vi "Plot Euler Spiral.vi"() -> ()   [LabVIEW 2018]
panel:
  out "L2":dbl
  out "Normalized":cluster{"Time":dbl, "Length":dbl, "Radius":dbl}
  out "Scaled":cluster{"Time":dbl, "Length":dbl, "Radius":dbl}
  in  "Y Positive":bool=TRUE
  in  "X Positive":bool=TRUE
  out "Length to Vertex":dbl
  in  "Scale Mag":dbl(slide)=1.096774193548387 scale=0.0..10.0
  out "Tangent angle (deg)":dbl
  in  "Additional circle arc (rad)":dbl(slide) scale=0.0..3.0
  out "Tangent angle (rad)":dbl
  out "Tangent Point":cluster{dbl, dbl}
  in  "Steps":dbl=1000.0
  in  "T":dbl(slide)=0.6451612903225806 scale=0.0..2.0
  out "XY Graph":cluster{cluster{dbl, dbl}[]}[](graph)
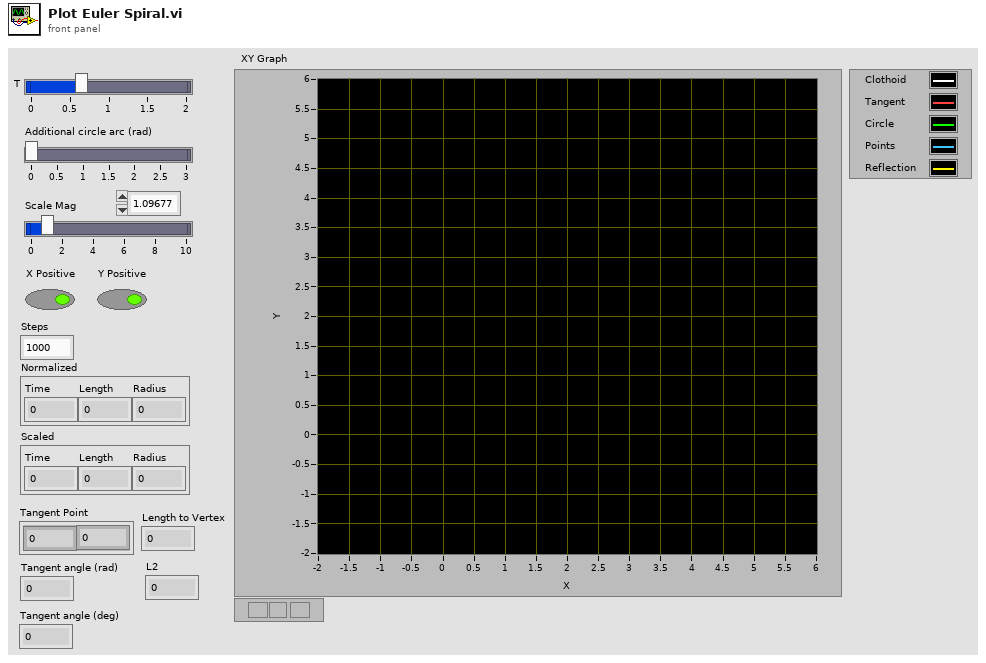
[diagram p1: front panel]
types:
  T1 = cluster{cluster{dbl, dbl}[], cluster{dbl, dbl}[], cluster{dbl, dbl}}
  T2 = cluster{"Negated Y":i32, "Scaled Sign Vector":cluster{"X":dbl, "Y":dbl}, "Combined":i32, "Additional circle arc (rad)":dbl}
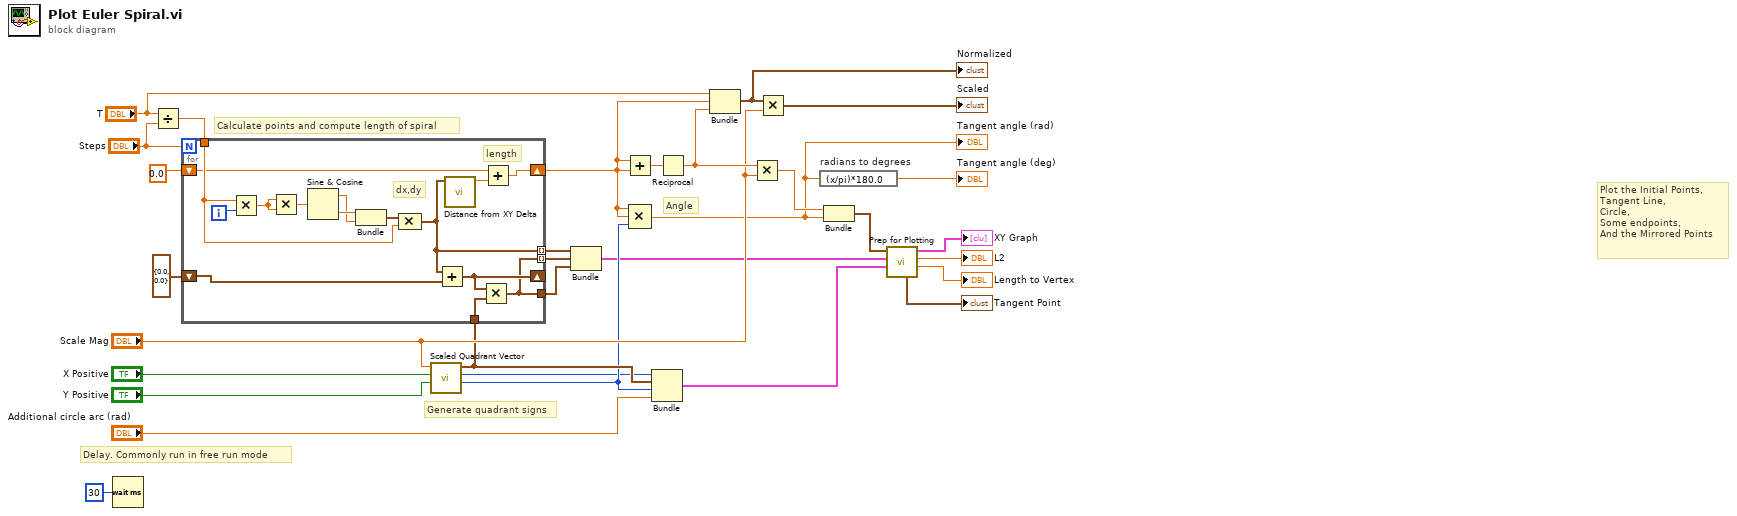
[diagram p0: block diagram]
diagram:
  # "Generate quadrant signs"
  # "Delay. Commonly run in free run mode"
  # "Plot the Initial Points,\nTangent Line,\nCircle,\nSome endpoints,\nAnd the Mirrored Points"
  # "Angle"
  # "Calculate points and compute length of spiral"
  n1 = Wait (ms)(milliseconds to wait=u32 30) -> ()  [unwired: 1 out]
  n2 = Divide(x="T", y="Steps") -> (x/y=w29:dbl)
  n3 = call "Scaled Quadrant Vector.vi"("Y Positive"="Y Positive", "X Positive"="X Positive", "Scale Mag"="Scale Mag") -> ("Combined"=w9:i32, "Negated Y"=w7:i32, "Scaled Sign Vector"=w10:cluster{"X":dbl, "Y":dbl})  [unwired: 6 in]
  n4 = for {
    N: "Steps" -> [_]
    shift-right: [w39] -> _
    shift-left: cluster{dbl, dbl} {0.0, 0.0} -> [w41]
    tunnel: [w32] -> w1 mode=indexing
    tunnel: w29 -> [w38]
    shift-right: [w35] -> w19
    shift-left: 0.0 -> [w37]
    tunnel: [w33] -> w3
    tunnel: [w33] -> w2 mode=indexing
    tunnel: w10 -> [w34]
    i -> [w46]
    # "length"
    # "dx,dy"
    n5 = Multiply(x=w38, y=w46) -> (x*y=w40:dbl)
    n6 = Multiply(x=w40, y=w40) -> (x*y=w45:dbl)
    n7 = Sine & Cosine(0:w45) -> (1:w43:dbl, 2:w44:dbl)
    n8 = Bundle(w44, w43) -> (w42:cluster{dbl, dbl})  [unwired: 1 in]
    n9 = Compound Arithmetic op=MULTIPLY(w42, w38) -> (w32:cluster{dbl, dbl})
    n10 = Add(x=w32, y=w41) -> (x+y=w39:cluster{dbl, dbl})
    n11 = call "Distance from XY Delta.vi"("Delta Point"=w32) -> ("Distance"=w36:dbl)  [unwired: 10 in]
    n12 = Multiply(x=w39, y=w34) -> (x*y=w33:cluster{dbl, dbl})
    n13 = Add(x=w37, y=w36) -> (x+y=w35:dbl)
  }
  n14 = Bundle(w1, w2, w3) -> (w5:T1)  [unwired: 1 in]
  n15 = Add(x=w19, y=w19) -> (x+y=w27:dbl)
  n16 = Compound Arithmetic op=MULTIPLY(w19, w19, w9) -> (w8:dbl)
  "Tangent angle (rad)" <- w8
  n17 = Bundle("Negated Y"=w7, "Scaled Sign Vector"=w10, "Combined"=w9, "Additional circle arc (rad)"="Additional circle arc (rad)") -> (w11:T2)  [unwired: 1 in]
  n18 = Reciprocal(x=w27) -> (1/x=w18:dbl)
  n19 = Bundle("T"="T", w19, w18) -> (w16:cluster{"T":dbl, dbl, dbl})  [unwired: 1 in]
  "Normalized" <- w16
  n20 = Multiply(x=w18, y="Scale Mag") -> (x*y=w12:dbl)
  n21 = Multiply(x=w16, y="Scale Mag") -> (x*y=→"Scaled":cluster{"T":dbl, dbl, dbl})
  n22 = expression code="(x/pi)*180.0" "radians to degrees"(w8) -> (→"Tangent angle (deg)":dbl)
  n23 = Bundle(w12, w8) -> (w13:cluster{dbl, dbl})  [unwired: 1 in]
  n24 = call "Prep for Plotting.vi"("Quad Info"=w11, "Points"=w5, "Circle Info"=w13) -> ("Length to Vertex"=→"Length to Vertex":dbl, "L2"=→"L2":dbl, "XY Graph"=→"XY Graph":cluster{"Array":cluster{dbl, dbl}[]}[], "Tangent Point"=→"Tangent Point":cluster{dbl, dbl})  [unwired: 5 in]
